vi "WorkorderHandler_Destroy.vi"(8 "error in (no error)":errorcluster, 11 "reference":T1) -> (0 "error out":errorcluster)   [LabVIEW 2011]
uses:
  DataStructures/WorkorderHandler_ObjectReference.ctl
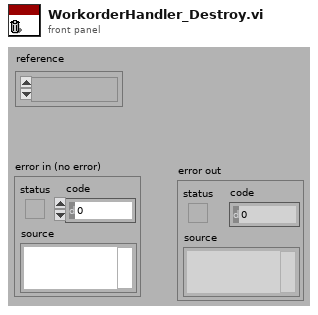
[diagram p1: front panel]
types:
  T1 = typedef "WorkorderHandler_ObjectReference.ctl" = refnum<k1>
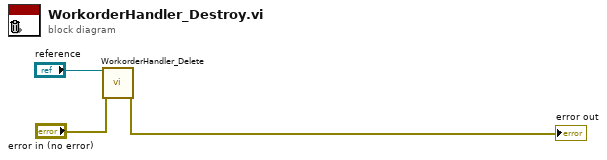
[diagram p0: block diagram]
diagram:
  n1 = call "WorkorderHandler_Delete.vi"("reference"="reference", "error in (no error)"="error in (no error)") -> ("error out"=→"error out":errorcluster)  [unwired: 1 in, 16 out]
